vi "5.10 Randy Buffers.vi"(1 "Randy":T2) -> (0 "Randy Buffers":T1)   [LabVIEW 2010]
uses:
  <vilib>/userDefined/High Color/IMAQdx.ctl
  5.10 Buffers Cluster.ctl
  <vilib>/vision/Image Controls.llb/IMAQ Image.ctl
  <vilib>/vision/driver/IMAQdx.llb/IMAQdx Camera Control Mode.ctl
  <vilib>/vision/driver/NI_Vision_Acquisition_Software.lvlib
  Program Files (x86)/National Instruments/LabVIEW 2010/resource/objmgr/imaqdx.rc
panel:
  out "EnumStrings[]":string[](array[string])
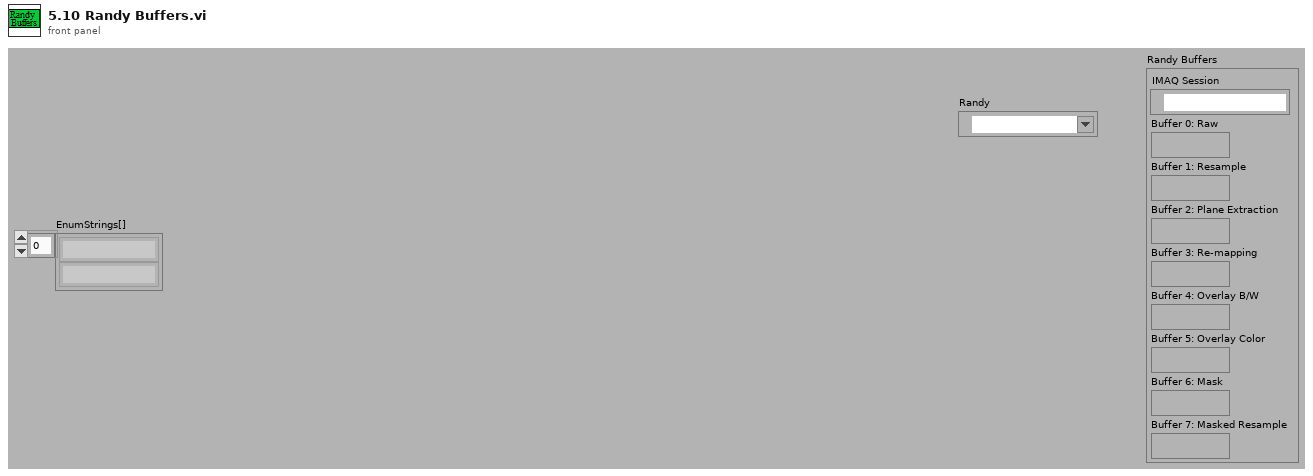
[diagram p1: front panel]
types:
  T1 = typedef "5.10 Buffers Cluster.ctl" = cluster{"IMAQ Session":T2, "Buffer 0: Raw":T3, "Buffer 1: Resample":T3, "Buffer 2: Plane Extraction":T3, "Buffer 3: Re-mapping":T3, "Buffer 4: Overlay B/W":T3, "Buffer 5: Overlay Color":T3, "Buffer 6: Mask":T3, "Buffer 7: Masked Resample":T3}
  T2 = typedef "IMAQdx.ctl" = refnum<k21>
  T3 = typedef "IMAQ Image.ctl" = refnum<image>
  T4 = typedef "Image Type" = u32
  T5 = typedef "NI_Vision_Acquisition_Software.lvlib/IMAQdx Camera Control Mode.ctl" = enum32{"Controller", "Listener"}
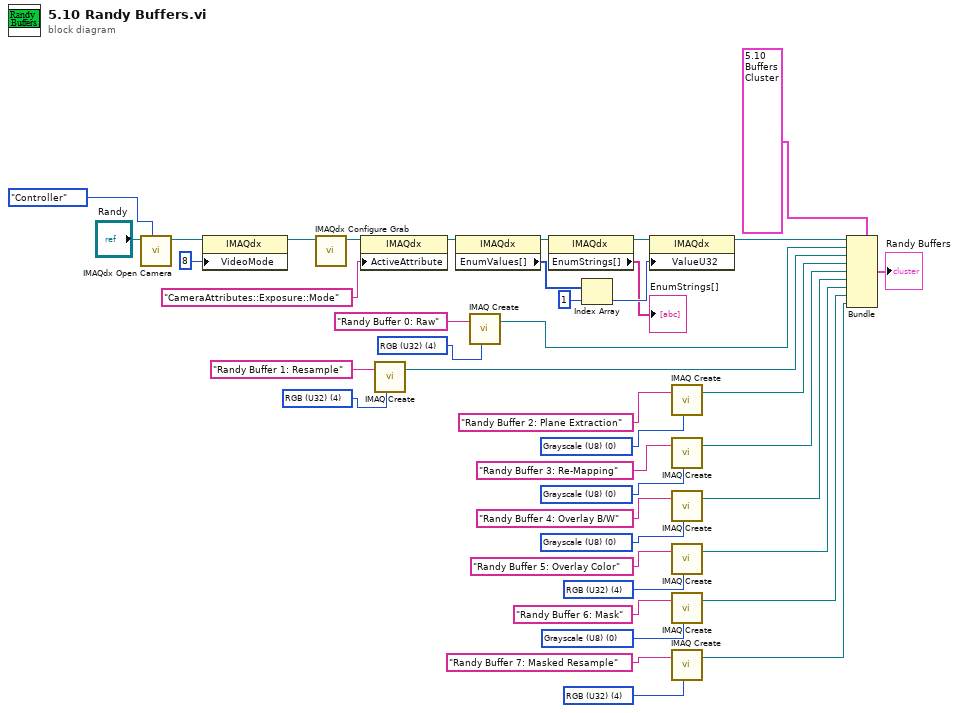
[diagram p0: block diagram]
diagram:
  w3 = T4 4 items=["Grayscale (U8)", "Grayscale (I16)", "Grayscale (SGL)", "Complex (CSG)", "RGB (U32)", "HSL (U32)", "RGB (U64)", "Grayscale (U16)"] ("Image Type")
  w6 = T4 0 items=["Grayscale (U8)", "Grayscale (I16)", "Grayscale (SGL)", "Complex (CSG)", "RGB (U32)", "HSL (U32)", "RGB (U64)", "Grayscale (U16)"] ("Image Type")
  w33 = T4 4 items=["Grayscale (U8)", "Grayscale (I16)", "Grayscale (SGL)", "Complex (CSG)", "RGB (U32)", "HSL (U32)", "RGB (U64)", "Grayscale (U16)"] ("Image Type")
  w25 = T4 0 items=["Grayscale (U8)", "Grayscale (I16)", "Grayscale (SGL)", "Complex (CSG)", "RGB (U32)", "HSL (U32)", "RGB (U64)", "Grayscale (U16)"] ("Image Type")
  w24 = T4 4 items=["Grayscale (U8)", "Grayscale (I16)", "Grayscale (SGL)", "Complex (CSG)", "RGB (U32)", "HSL (U32)", "RGB (U64)", "Grayscale (U16)"] ("Image Type")
  w21 = T4 4 items=["Grayscale (U8)", "Grayscale (I16)", "Grayscale (SGL)", "Complex (CSG)", "RGB (U32)", "HSL (U32)", "RGB (U64)", "Grayscale (U16)"] ("Image Type")
  w20 = T4 0 items=["Grayscale (U8)", "Grayscale (I16)", "Grayscale (SGL)", "Complex (CSG)", "RGB (U32)", "HSL (U32)", "RGB (U64)", "Grayscale (U16)"] ("Image Type")
  w17 = T4 0 items=["Grayscale (U8)", "Grayscale (I16)", "Grayscale (SGL)", "Complex (CSG)", "RGB (U32)", "HSL (U32)", "RGB (U64)", "Grayscale (U16)"] ("Image Type")
  n1 = call <vilib>:"IMAQdx Open Camera.vi"("Camera Control Mode"=IMAQdx_Camera_Control_Mode."Controller", "Session In"="Randy") -> ("Session Out"=w29:T2)  [unwired: 8 in, 1 out]
  n2 = property class="IMAQdx"(reference=w29, "VideoMode"=u32 8) -> (reference out=w31:T2)  [unwired: 1 in, 1 out]
  n3 = call <vilib>:"IMAQdx Configure Grab.vi"("Session In"=w31) -> ("Session Out"=w8:T2)  [unwired: 9 in, 1 out]
  n4 = property class="IMAQdx"(reference=w8, "ActiveAttribute"="CameraAttributes::Exposure::Mode") -> (reference out=w15:T2)  [unwired: 1 in, 1 out]
  n5 = call "IMAQ Create"("Image Name"="Randy Buffer 1: Resample", "Image Type"=w24) -> ("New Image"=w35:T3)  [unwired: 3 in, 1 out]
  n6 = property class="IMAQdx"(reference=w15) -> (reference out=w11:T2, "EnumValues[]"=w14:u32[])  [unwired: 1 in, 1 out]
  n7 = call "IMAQ Create"("Image Name"="Randy Buffer 0: Raw", "Image Type"=w33) -> ("New Image"=w34:T3)  [unwired: 3 in, 1 out]
  n8 = property class="IMAQdx"(reference=w11) -> (reference out=w10:T2, "EnumStrings[]"=→"EnumStrings[]":string[])  [unwired: 1 in, 1 out]
  n9 = Index Array(array=w14, index=u32 1 ("ValueU32")) -> (element=w12:u32)
  n10 = property class="IMAQdx"(reference=w10, "ValueU32"=w12) -> (reference out=w7:T2)  [unwired: 1 in, 1 out]
  n11 = call "IMAQ Create"("Image Name"="Randy Buffer 2: Plane Extraction", "Image Type"=w25) -> ("New Image"=w36:T3)  [unwired: 3 in, 1 out]
  n12 = call "IMAQ Create"("Image Name"="Randy Buffer 3: Re-Mapping", "Image Type"=w20) -> ("New Image"=w37:T3)  [unwired: 3 in, 1 out]
  n13 = call "IMAQ Create"("Image Name"="Randy Buffer 4: Overlay B/W", "Image Type"=w17) -> ("New Image"=w38:T3)  [unwired: 3 in, 1 out]
  n14 = call "IMAQ Create"("Image Name"="Randy Buffer 5: Overlay Color", "Image Type"=w21) -> ("New Image"=w39:T3)  [unwired: 3 in, 1 out]
  n15 = call "IMAQ Create"("Image Name"="Randy Buffer 6: Mask", "Image Type"=w6) -> ("New Image"=w2:T3)  [unwired: 3 in, 1 out]
  n16 = call "IMAQ Create"("Image Name"="Randy Buffer 7: Masked Resample", "Image Type"=w3) -> ("New Image"=w1:T3)  [unwired: 3 in, 1 out]
  n17 = Bundle(cluster=T1 {"IMAQ Session"="", "Buffer 0: Raw"=refnum, "Buffer 1: Resample"=refnum, "Buffer 2: Plane Extraction"=refnum, "Buffer 3: Re-mapping"=refnum, "Buffer 4: Overlay B/W"=refnum, "Buffer 5: Overlay Color"=refnum, "Buffer 6: Mask"=refnum, "Buffer 7: Masked Resample"=refnum} ("output cluster"), "IMAQ Session"=w7, "Buffer 0: Raw"=w34, "Buffer 1: Resample"=w35, "Buffer 2: Plane Extraction"=w36, "Buffer 3: Re-mapping"=w37, "Buffer 4: Overlay B/W"=w38, "Buffer 5: Overlay Color"=w39, "Buffer 6: Mask"=w2, "Buffer 7: Masked Resample"=w1) -> (→"Randy Buffers":T1)
